vi "FPGA_SystemAsynch VI Registration.vi"(10 "Operation":enum16{"Get", "Add", "Remove"}(ring), 11 "VI Refnum":refnum<vi>) -> (3 "VI Refs":refnum<vi>[](array[refnum]))   [LabVIEW 2017]
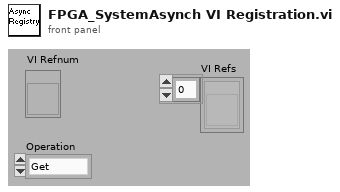
[diagram p1: front panel]
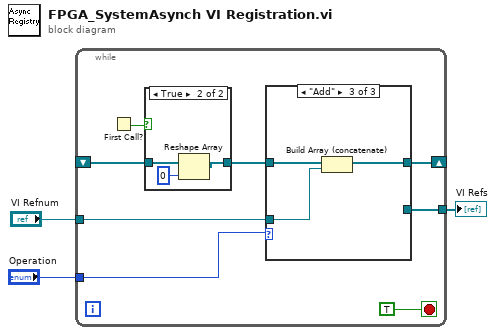
[diagram p0: block diagram]
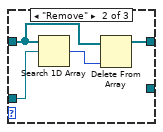
[diagram p3: hidden frame]
diagram:
  n1 = while {
    shift-right: [w8] -> _
    shift-left: _ -> [w9]
    tunnel: "VI Refnum" -> [w5]
    tunnel: "Operation" -> [w6]
    tunnel: [w4] -> w1
    stop <- TRUE stop-if-true
    n2 = First Call?() -> (First Call?: T/F=w10:bool)
    n3 = case shown="True" w10 {
      tunnel: w9 -> [w20 w23]
      tunnel: [w20 w22] -> w7
      frame False {
      }
      frame True {
        n4 = Reshape Array(w23, 0 ("dimension size")) -> (w22:refnum<vi>[])
      }
    }
    n5 = case shown="\"Add\"" w6 {
      tunnel: [w12 w13 w18] -> w8
      tunnel: w7 -> [w12 w14 w19]
      tunnel: w5 -> [_ w16 w17]
      tunnel: [w12 _ _] -> w4
      frame "Get", Default {
      }
      frame "Remove" {
        n6 = Search 1D Array(1D array=w14, element=w16) -> (index of element=w15:i32)  [unwired: 1 out]
        n7 = Delete From Array(array=w14, index=w15) -> (array with subset deleted=w13:refnum<vi>[])  [unwired: 1 in, 1 out]
      }
      frame "Add" {
        n8 = Build Array (concatenate)(w19, w17) -> (w18:refnum<vi>[])
      }
    }
  }
  "VI Refs" <- w1
